vi "Speed_PI_Control_Sim.vi"(6 "Speed":dbl, 7 "Speed Ki":dbl(slide)=10.0 scale=1.0..10.0, 8 "Slope Gain":dbl, 9 "Desired_Speed":dbl, 10 "Speed Kp":dbl(slide)=0.49679802955665026 scale=0.1..1.0, 11 "slope":dbl) -> (2 "Vm":dbl)   [LabVIEW 2018]
uses:
  <vilib>/Simulation/Implementation/Shared/SIMSCR Execution Mode.ctl
  <vilib>/Simulation/Scripting/Companion Diagram/SimConfigNode/SimParams.ctl
  <vilib>/Simulation/Scripting/Companion Diagram/SimConfigNode/_simSolvers.ctl
  <vilib>/Simulation/Param Hierarchy/Typedefs/SIMPH Param Control Actions.ctl
  <vilib>/Simulation/Implementation/Shared/SIM limit type.ctl
  <vilib>/Simulation/Implementation/Shared/NILVSim_ParamChanged.vi
  <vilib>/Simulation/Implementation/Shared/NILVSIM_BeginStep.vi
  <vilib>/Simulation/SignalArithmetic/Implementation/NILVSim Gain.llb/SIM Gain (scalar).vi
  <vilib>/Simulation/Nonlinear/Implementation/NILVSim Saturation.llb/SIM Saturation (scalar).vi
  <vilib>/Simulation/ContinuousLinear/Implementation/NILVSim Integrator new.llb/SIM Integrator distributor (scalar).vi
  <vilib>/Simulation/ContinuousLinear/Implementation/NILVSim Integrator new.llb/SIM Integrator collector (scalar).vi
  <vilib>/Simulation/Implementation/Shared/NILVSim_Manager.vi
  <vilib>/Utility/error.llb/Clear Errors.vi
  <vilib>/Simulation/Implementation/Shared/NILVSim_FinalizeModel.vi
  <vilib>/Simulation/Implementation/Shared/SIM Unbundle Sim Info.vi
  <vilib>/Simulation/Implementation/Shared/SIMSH Read Queue.vi
  <vilib>/Simulation/Implementation/Shared/NILVSim_Initialize.vi
  <vilib>/Simulation/Utility/Implementation/NILVSim Get Time and IsAcceptedStep.vi
  <vilib>/Simulation/Implementation/Shared/NILVSim_GetModelError.vi
  <vilib>/Simulation/Implementation/Shared/SIM SimErrorHandler.vi
  <vilib>/Simulation/Implementation/Shared/SIM Bundle Sim Info.vi
  <vilib>/Simulation/Scripting/Companion Diagram/SimConfigNode/SimDog.xnode
  <vilib>/Simulation/Implementation/XNodeFramework/SimXNode/SimX.xnode
  <vilib>/Simulation/ContinuousLinear/Implementation/NILVSim Integrator new.llb/SIM Integrator (scalar).vi
  <vilib>/Simulation/Implementation/Shared/NI_SIM_Implementation.lvlib
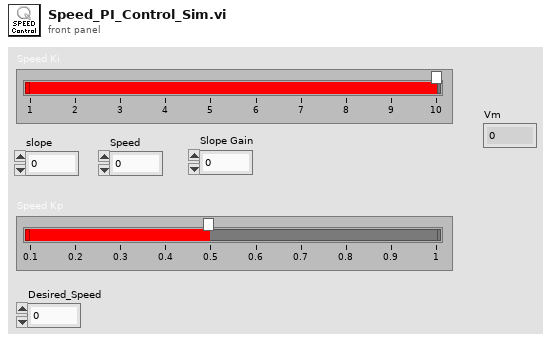
[diagram p1: front panel]
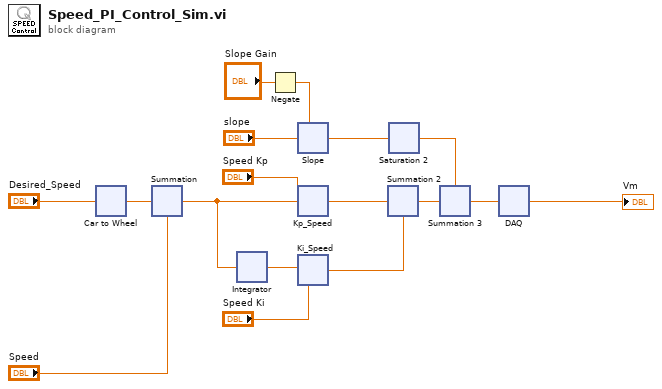
[diagram p0: block diagram]
diagram:
  n1 = xnode "Car to Wheel"("input"="Desired_Speed") -> ("output"=w15:dbl)  [unwired: 3 in]
  n2 = xnode ("Summation")("Operand1"=w15, "Operand2"="Speed") -> ("Result"=w7:dbl)
  n3 = xnode "Integrator"("input"=w7) -> ("output"=w8:dbl)  [unwired: 9 in, 2 out]
  n4 = Negate(x="Slope Gain") -> (-x=w2:dbl)
  n5 = xnode "Slope"("gain"=w2, "input"="slope") -> ("output"=w11:dbl)  [unwired: 2 in]
  n6 = xnode ("Kp_Speed")("gain"="Speed Kp", "input"=w7) -> ("output"=w6:dbl)  [unwired: 2 in]
  n7 = xnode ("Ki_Speed")("gain"="Speed Ki", "input"=w8) -> ("output"=w9:dbl)  [unwired: 2 in]
  n8 = xnode ("Summation 2")("Operand1"=w6, "Operand2"=w9) -> ("Result"=w10:dbl)
  n9 = xnode ("Saturation 2")("input"=w11) -> ("output"=w12:dbl)  [unwired: 4 in]
  n10 = xnode ("Summation 3")("Operand1"=w12, "Operand2"=w10) -> ("Result"=w5:dbl)
  n11 = xnode "DAQ"("input"=w5) -> ("output"=→"Vm":dbl)  [unwired: 4 in]
